vi "Read ALR_index.vi"(11 "Heater in":refnum<class "Heater.lvclass">) -> (2 "ALR_index":i32[](array[numeric]), 3 "Heater out":refnum<class "Heater.lvclass">)   [LabVIEW 2019, in "Heating.lvlib" / "Heater.lvclass"]
uses:
  Heater.lvclass
  Heater.lvclass/Heater.ctl
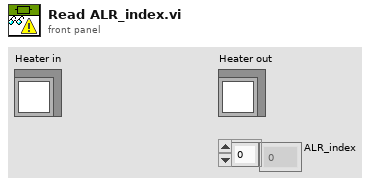
[diagram p1: front panel]
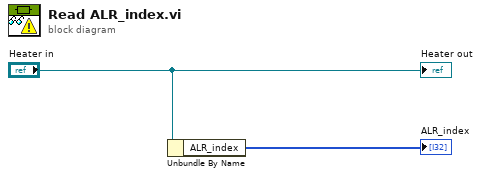
[diagram p0: block diagram]
diagram:
  n1 = Unbundle By Name("Heater in") -> ("ALR_index"=→"ALR_index":i32[])
  "Heater out" <- "Heater in"
